vi "File.Async Mover.vi"(9 "Error Msg":T1={"Cmd"="Task", "Sub"="Warning", "Data1"=variant, "Data2"=variant}, 10 "Parent Q":refnum<queue>, 11 "Q Name":string="FileMover") -> ()   [LabVIEW 2018]
uses:
  <vilib>/KATE/Queues/Q.Element.ctl
  File.Async Mover Move Task Item.ctl
  Errors/Error.Error Code List.ctl
  <vilib>/KATE/Queues/Queue Utils.lvlib
  <vilib>/KATE/Files/File Utils.lvlib
  <vilib>/KATE/Scheduler/Scheduler.lvlib
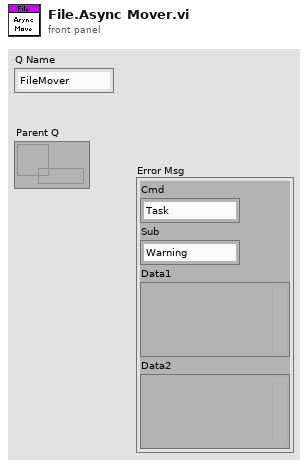
[diagram p1: front panel]
types:
  T1 = typedef "KATE_Lib.lvlib/Queue Utils.lvlib/Q.Element.ctl" = cluster{"Cmd":string, "Sub":string, "Data1":variant, "Data2":variant}
  T2 = typedef "File.Async Mover Move Task Item.ctl" = cluster{"Source":path, "DestDir":path, "DestSuffix":string, "Action":enum16{"Move", "Copy"}}
  T3 = typedef "Error.Error Code List.ctl" = i32
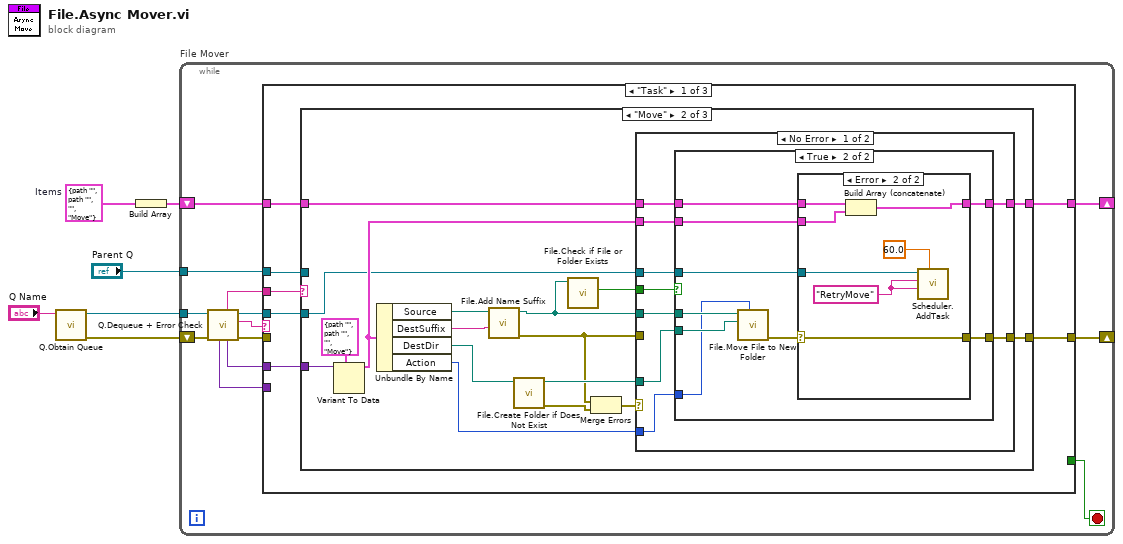
[diagram p0: block diagram]
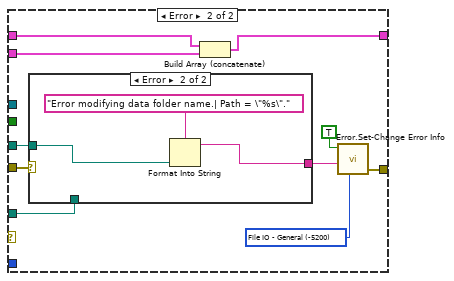
[diagram p5: hidden frame]
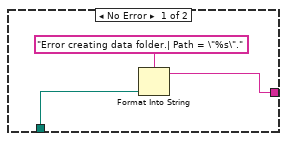
[diagram p6: hidden frame]
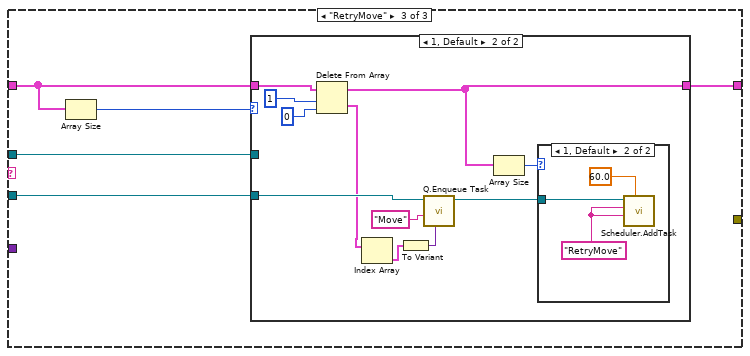
[diagram p7: hidden frame]
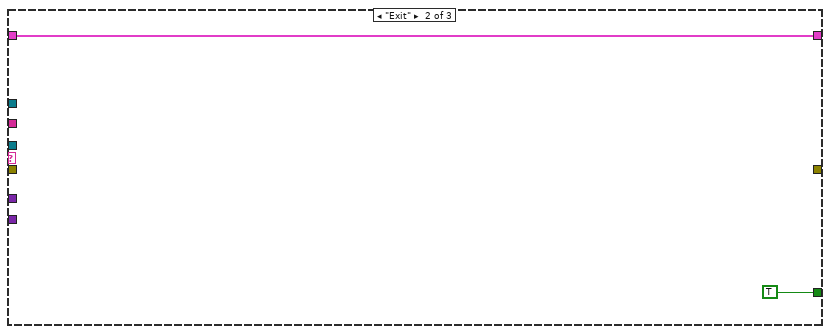
[diagram p10: hidden frame]
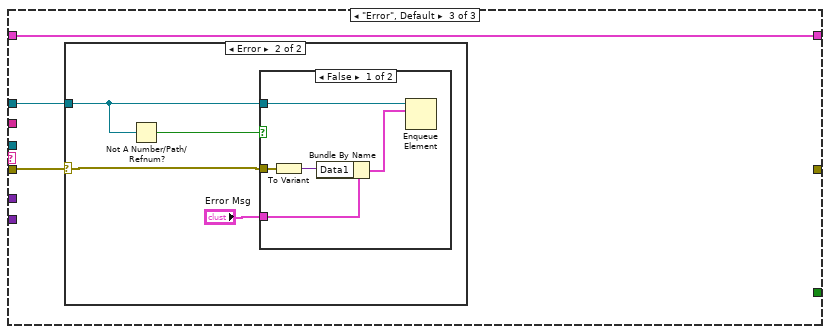
[diagram p11: hidden frame]
diagram:
  w1 = T2 {"Source"=path "", "DestDir"=path "", "DestSuffix"="", "Action"=enum."Move"}  # Items
  n1 = call <vilib>:"Q.Obtain Queue.vi"("Q Name"="Q Name") -> ("error out"=w6:errorcluster, "Q Out"=w5:refnum<queue>)  [unwired: 8 in, 1 out]
  n2 = Build Array(w1) -> (w2:T2[])
  n3 = while "File Mover" {
    tunnel: w5 -> [w19]
    shift-right: [w14] -> _
    shift-left: w6 -> [w18]
    tunnel: "Parent Q" -> [w12]
    shift-right: [w8] -> _
    shift-left: w2 -> [w9]
    stop <- w11 stop-if-true
    n4 = call <vilib>:"Q.Dequeue + Error Check.vi"("Error In"=w18, "Q In"=w19) -> ("error out"=w10:errorcluster, "Cmd"=w13:string, "Q Out"=w17:refnum<queue>, "Data1"=w16:variant, "Sub"=w7:string, "Data2"=w15:variant)  [unwired: 4 in]
    n5 = case shown="\"Task\"" w13 {
      tunnel: w17 -> [w20 _ _]
      tunnel: w16 -> [w26 _ _]
      tunnel: w15 -> [_ _ _]
      tunnel: [w23 _ _] -> w14
      tunnel: w12 -> [w21 _ w111]
      tunnel: [_ TRUE _] -> w11
      tunnel: w10 -> [_ _ w112]
      tunnel: w9 -> [w25 w108 w110]
      tunnel: [w24 w108 w110] -> w8
      tunnel: w7 -> [w22 _ _]
      frame "Task" {
        n6 = case shown="\"Move\"" w22 {
          tunnel: w26 -> [_ w44 _]
          tunnel: w25 -> [w27 w42 w91]
          tunnel: [w27 w41 w90] -> w24
          tunnel: [_ w39 _] -> w23
          tunnel: w21 -> [_ _ w89]
          tunnel: w20 -> [_ w38 w88]
          frame Default {
          }
          frame "Move" {
            n7 = Variant To Data(type=T2 {"Source"=path "", "DestDir"=path "", "DestSuffix"="", "Action"=enum."Move"} ("cluster"), Variant=w44) -> (data=w40:T2)  [unwired: 1 in, 1 out]
            n8 = Unbundle By Name(w40) -> ("Source"=w34:path, "DestSuffix"=w33:string, "DestDir"=w35:path, "Action"=w28:enum16{"Move", "Copy"})
            n9 = call "File.Add Name Suffix.vi"("DestSuffix"=w33, "Source"=w34) -> ("error out"=w29:errorcluster, "New Path"=w32:path)  [unwired: 8 in]
            n10 = call <vilib>:"File.Create Folder if Does Not Exist.vi"("Path"=w35) -> ("error out"=w30:errorcluster, "Dup Path"=w36:path)  [unwired: 8 in, 1 out]
            n11 = call <vilib>:"File.Check if File or Folder Exists.vi"("Path"=w32) -> ("Exists"=w43:bool)  [unwired: 6 in, 4 out]
            n12 = Merge Errors(w29, w30) -> (w31:errorcluster)
            n13 = case shown="No Error" w31 {
              tunnel: w32 -> [w53 w72]
              tunnel: w43 -> [w52 _]
              tunnel: w42 -> [w51 w77]
              tunnel: [w50 w75] -> w41
              tunnel: w40 -> [w49 w76]
              tunnel: [w48 w78] -> w39
              tunnel: w38 -> [w47 _]
              tunnel: w36 -> [w46 w74]
              tunnel: w29 -> [_ w73]
              tunnel: w28 -> [w45 _]
              frame No Error {
                n14 = case shown="True" w52 {
                  tunnel: w46 -> [_ w56]
                  tunnel: w53 -> [_ w57]
                  tunnel: w51 -> [w54 w62]
                  tunnel: [w54 w61] -> w50
                  tunnel: w49 -> [_ w60]
                  tunnel: [_ w59] -> w48
                  tunnel: w47 -> [_ w58]
                  tunnel: w45 -> [_ w55]
                  frame False {
                    # "Do Nothing"
                  }
                  frame True {
                    n15 = call "File.Move File to New Folder.vi"("Action"=w55, "Destination Folder"=w56, "Source File Path"=w57) -> ("error out"=w63:errorcluster)  [unwired: 7 in, 1 out]
                    n16 = case shown="Error" w63 {
                      selector: w63 -> [_ w68]
                      tunnel: w62 -> [w64 w71]
                      tunnel: [w64 w70] -> w61
                      tunnel: w60 -> [_ w69]
                      tunnel: [_ w68] -> w59
                      tunnel: w58 -> [_ w67]
                      frame No Error {
                      }
                      frame Error {
                        w65 = "RetryMove"
                        n17 = Build Array (concatenate)(w71, w69) -> (w70:T2[])
                        n18 = call <vilib>:"Scheduler.AddTask.vi"("Interval(s)"=60.0, "Task Name"=w65, "Sched Name"=w65, "Q In"=w67) -> ()  [unwired: 6 in, 2 out]
                      }
                    }
                  }
                }
              }
              frame Error {
                w80 = T3 -5200 items=["No Error"=0, "Abort"=-2, "Misc"=-5000, "Fixture Error"=-5100, "File IO - General"=-5200, "FIle IO - Config Error"=-5201, "Instrument - General"=-5300, "Instrument - Serial Com"=-5301, "Instrument - Camera"=-5302, "Instrument - PS"=-5303, "Instrument - Oscilloscope"=-5304, "Instrument - Function Gen"=-5305, "Instrument - Load"=-5306, "Instrument - Meter"=-5307, "Instrument - Power Control"=-5308, "Instrument - Motion"=-5309, "Instrument - RF"=-5310, "System Exe"=-5400, "Image Processing"=-5500, "Communication"=-5600, "Script - Syntax Error"=-6000, "Script - Invalid Name or Param"=-6100, "Script - Timeout"=-6200, "Invalid Data"=-6300, "FW Update Error"=-6500] ("Std Code")
                n19 = case shown="Error" w73 {
                  tunnel: [w83 w86] -> w79
                  tunnel: w74 -> [w82 _]
                  tunnel: w72 -> [_ w85]
                  frame No Error {
                    n20 = Format Into String(format string="Error creating data folder.| Path = \"%s\".", w82) -> (resulting string=w83:string)  [unwired: 2 in, 1 out]
                  }
                  frame Error {
                    n21 = Format Into String(format string="Error modifying data folder name.| Path = \"%s\".", w85) -> (resulting string=w86:string)  [unwired: 2 in, 1 out]
                  }
                }
                n22 = Build Array (concatenate)(w77, w76) -> (w75:T2[])
                n23 = call "Error.Set-Change Error Info.vi"("Std Code"=w80, "Description"=w79, "Set Error"=TRUE) -> ("error out"=w78:errorcluster)  [unwired: 8 in]
              }
            }
          }
          frame "RetryMove" {
            n24 = Array Size(array=w91) -> (size(s)=w92:i32)
            n25 = case shown="1, Default" w92 {
              tunnel: w91 -> [w93 w104]
              tunnel: [w93 w98] -> w90
              tunnel: w89 -> [_ _]
              tunnel: w88 -> [_ w96]
              frame 0 {
                # "Do Nothing"
              }
              frame 1, Default {
                n26 = Delete From Array(array=w104, length=1, index=0) -> (deleted portion=w95:T2[], array with subset deleted=w98:T2[])
                n27 = Index Array(array=w95) -> (element=w94:T2)  [unwired: 1 in]
                n28 = To Variant(anything=w94) -> (Variant=w101:variant)
                n29 = call <vilib>:"Q.Enqueue Task.vi"("Data1"=w101, "Task Name"="Move", "Q In"=w96) -> ("Q Out"=w99:refnum<queue>)  [unwired: 7 in, 1 out]
                n30 = Array Size(array=w98) -> (size(s)=w97:i32)
                n31 = case shown="1, Default" w97 {
                  tunnel: w99 -> [_ w105]
                  frame 0 {
                  }
                  frame 1, Default {
                    w106 = "RetryMove"
                    n32 = call <vilib>:"Scheduler.AddTask.vi"("Interval(s)"=60.0, "Task Name"=w106, "Sched Name"=w106, "Q In"=w105) -> ()  [unwired: 6 in, 2 out]
                  }
                }
              }
            }
          }
        }
      }
      frame "Exit" {
        (unwired) TRUE
      }
      frame "Error", Default {
        n33 = case shown="Error" w112 {
          selector: w112 -> [_ w113]
          tunnel: w111 -> [_ w115]
          frame No Error {
          }
          frame Error {
            n34 = Not A Number/Path/Refnum?(number/path/refnum=w115) -> (NaN/Path/Refnum?=w116:bool)
            n35 = case shown="False" w116 {
              tunnel: w115 -> [w121 _]
              tunnel: "Error Msg" -> [w120 _]
              tunnel: w113 -> [w117 _]
              frame False {
                n36 = To Variant(anything=w117) -> (Variant=w118:variant)
                n37 = Bundle By Name(cluster=w120, "Data1"=w118) -> (w119:T1)
                n38 = Enqueue Element(queue=w121, element=w119) -> ()  [unwired: 2 in, 3 out]
              }
              frame True {
              }
            }
          }
        }
      }
    }
  }
